vi "Main.vi"(11 "Module Admin":refnum<class "Delacor_lib_QMH_Module Admin.lvclass">) -> ()   [LabVIEW 2020, in "Navigation.lvlib"]
doc: "This template is based off of the Queued Message Handler design pattern and the Queued Message Handler project template that ships with LabVIEW.\n\nThe main difference is that the queue is private to this module and communication between modules is performed via Broadcast and Request events.\n\nRequest events are wrapped in public API methods and are handled in the Event Handling Loop (EHL) of this VI. Any module can register for Broadcast events sent by this module. The EHL generates messages based on user interface actions.\n\nThe Message Handling Loop (MHL) processes messages generated by the EHL, or by other messages. The messages are string values, so new messages can be added easily to the Message Cases case structure in the MHL. Each message cluster can also provide an optional value for Message Data, which is a variant that can be converted to whatever message-specific data is required.\n____\nHAMPEL SOFTWARE ENGINEERING v2.6.0 (2023-12-19 10:54)"
uses:
  Navigation.lvlib
  <vilib>/Delacor/Delacor QMH/Libraries/Module Admin_class/Delacor_lib_QMH_Module Admin.lvclass
  Button Manager/Control Refs.ctl
  Module Data--cluster.ctl
  <vilib>/Hampel Software Engineering/HSE Layout Manager/HSE Layout/HSE VBoxLayout/HSE VBoxLayout.lvclass
  Button Manager/Button Manager.lvclass
  Stop Argument--cluster.ctl
  <vilib>/Delacor/Delacor QMH/Libraries/Message Queue_class/Delacor_lib_QMH_Message Queue.lvclass/Delacor_lib_QMH_Message Queue.ctl
  <vilib>/Delacor/Delacor QMH/Libraries/Module Admin_class/Delacor_lib_QMH_Module Admin.lvclass/Delacor_lib_QMH_Module Admin.ctl
  Configure Argument--cluster.ctl
  Prepare Argument--cluster.ctl
  Update Navigation Argument--cluster.ctl
  Sub-VIs/Ctl Target.ctl
  Sub-VIs/ListBox Event Data.ctl
  Select Listbox Element Argument--cluster.ctl
  Set Visibility Argument--cluster.ctl
  Sub-VIs/Visibility options--enum.ctl
  Set Disabled State Argument--cluster.ctl
  Libraries/hse-libraries/Source/hse-application/hse-application.lvclass/hse-application.ctl
  Libraries/hse-libraries/Source/hse-dqmh/Controls/Module Display Scenarios.ctl
  <vilib>/Delacor/Delacor QMH/Libraries/Message Queue_class/Delacor_lib_QMH_Enqueue Message (Single).vi
  <vilib>/Delacor/Delacor QMH/Libraries/Module Admin_class/Delacor_lib_QMH_Get External Launch.vi
  Libraries/hse-libraries/Source/hse-application/HSE Application not initialized--error.vi
  Libraries/hse-libraries/Source/hse-application/hse-application__GetSingleton.vi
  <vilib>/Utility/sysdir.llb/Get System Directory.vi
  <vilib>/Utility/error.llb/Error Cluster From Error Code.vi
  <vilib>/ErrorRing/Error Ring.xnode
  <vilib>/Delacor/Delacor QMH/Libraries/Message Queue_class/Delacor_lib_QMH_Message Queue.lvclass
  Libraries/hse-libraries/Source/hse-configuration/config-ini/config-ini.lvclass
  Libraries/hse-libraries/Source/hse-application/hse-application.lvclass
  <vilib>/Hampel Software Engineering/HSE Logger/hse-logger.lvlib
  Libraries/hse-libraries/Source/hse-dqmh/hse-dqmh.lvlib
panel:
  in  "lb_sub_8":i32(listbox)
  in  "lb_sub_7":i32(listbox)
  in  "lb_sub_6":i32(listbox)
  in  "lb_sub_5":i32(listbox)
  in  "lb_sub_4":i32(listbox)
  in  "lb_sub_3":i32(listbox)
  in  "lb_sub_2":i32(listbox)
  in  "lb_sub_9":i32(listbox)
  in  "lb_sub_1":i32(listbox)
  in  "btn_top_9":bool
  in  "btn_top_8":bool
  in  "btn_top_7":bool
  in  "btn_top_6":bool
  in  "lb_sub_0":i32(listbox)
  in  "btn_top_5":bool
  in  "btn_top_4":bool
  in  "btn_top_3":bool
  in  "btn_top_2":bool
  in  "btn_top_1":bool
  in  "btn_top_0":bool
  out "error out":errorcluster
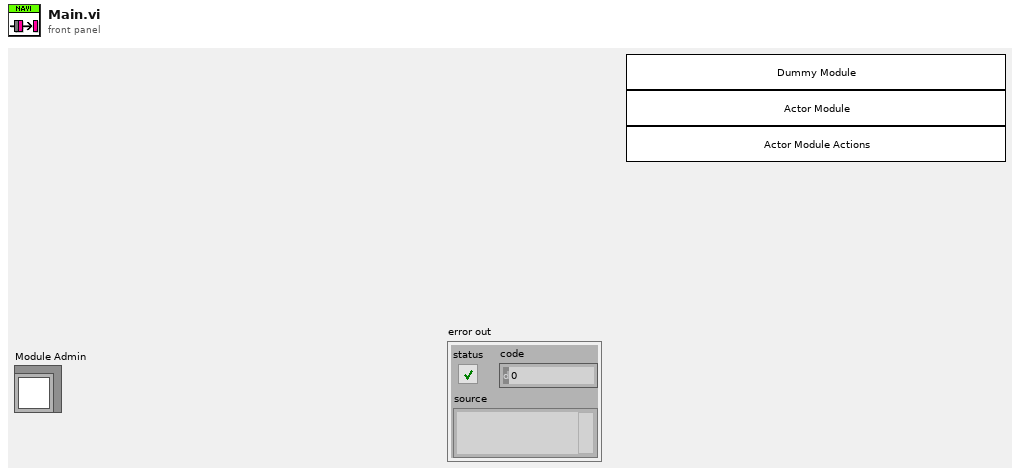
[diagram p1: front panel]
types:
  T1 = typedef "Navigation.lvlib/Button Manager.lvclass/Control Refs.ctl" = cluster{"Top Ctls":refnum<vi>[], "Sub Ctls":refnum<vi>[]}
  T2 = typedef "Navigation.lvlib/Request Events--cluster.ctl" = cluster{"Stop Module":refnum<user-event>, "Show Panel":refnum<user-event>, "Hide Panel":refnum<user-event>, "Get Module Execution Status":refnum<user-event>, "Show Diagram":refnum<user-event>, "Prepare":refnum<user-event>, "Update Navigation":refnum<user-event>, "Configure":refnum<user-event>, "Select Listbox Element":refnum<user-event>, "Set Visibility":refnum<user-event>, "Set Disabled State":refnum<user-event>}
  T3 = typedef "Navigation.lvlib/Module Data--cluster.ctl" = cluster{"VBox Layout":refnum<class "HSE VBoxLayout.lvclass">, "Button Manager":refnum<class "Button Manager.lvclass">, "Buttons Def File":path, "Subpanel VI Ref":refnum<vi>}
  T4 = enum32{"invalid lock state", "Not Locked", "Locked (No Password)", "Password-protected"}
  T5 = typedef "Navigation.lvlib/Stop Argument--cluster.ctl" = cluster{"Origin":string, "Exit via Stop Module Req?":bool, "Wait for Module to stop?":bool}
  T6 = typedef "Navigation.lvlib/Configure Argument--cluster.ctl" = cluster{"Boolean":bool}
  T7 = typedef "Navigation.lvlib/Prepare Argument--cluster.ctl" = cluster{"Boolean":bool}
  T8 = typedef "Navigation.lvlib/Update Navigation Argument--cluster.ctl" = cluster{"Ctl Target":T9, "Name":string, "Data":variant}
  T9 = typedef "Navigation.lvlib/Ctl Target.ctl" = enum16{"Top Button", "Sub ListBox"}
  T10 = typedef "Navigation.lvlib/ListBox Event Data.ctl" = cluster{"CtlRef":refnum<vi>, "NewVal":i32, "OldVal":i32}
  T11 = typedef "Navigation.lvlib/Select Listbox Element Argument--cluster.ctl" = cluster{"Name":string, "Index":i32}
  T12 = typedef "Navigation.lvlib/Set Visibility Argument--cluster.ctl" = cluster{"Control Name":string, "Visibility":T13}
  T13 = typedef "Navigation.lvlib/Visibility options--enum.ctl" = enum16{"visible", "hidden"}
  T14 = typedef "Navigation.lvlib/Set Disabled State Argument--cluster.ctl" = cluster{"Control Name":string, "Control State":enum8{"Enabled", "Disabled", "Disabled and Grayed Out"}}
  T15 = enum32{"Invalid", "Standard", "Closed", "Hidden", "Minimized", "Maximized"}
  T16 = typedef "hse-dqmh.lvlib/Module Display Scenarios.ctl" = enum16{"Stand-Alone", "Managed"}
  T17 = enum8{"Enabled", "Disabled", "Disabled and Grayed Out"}
  T18 = typedef "hse-dqmh.lvlib/System Message Source.ctl" = enum16{"module", "application", "network"}
  T19 = typedef "Navigation.lvlib/Button Manager.lvclass/Top Control.ctl" = cluster{"name":string, "caption":string, "tooltip":string, "enabled_state":string, "action":string, "display_scenario":string, "sub":T20[]}
  T20 = typedef "Navigation.lvlib/Button Manager.lvclass/Sub Control.ctl" = cluster{"name":string, "tooltip":string, "enabled_state":string, "content":string[], "retain value":bool}
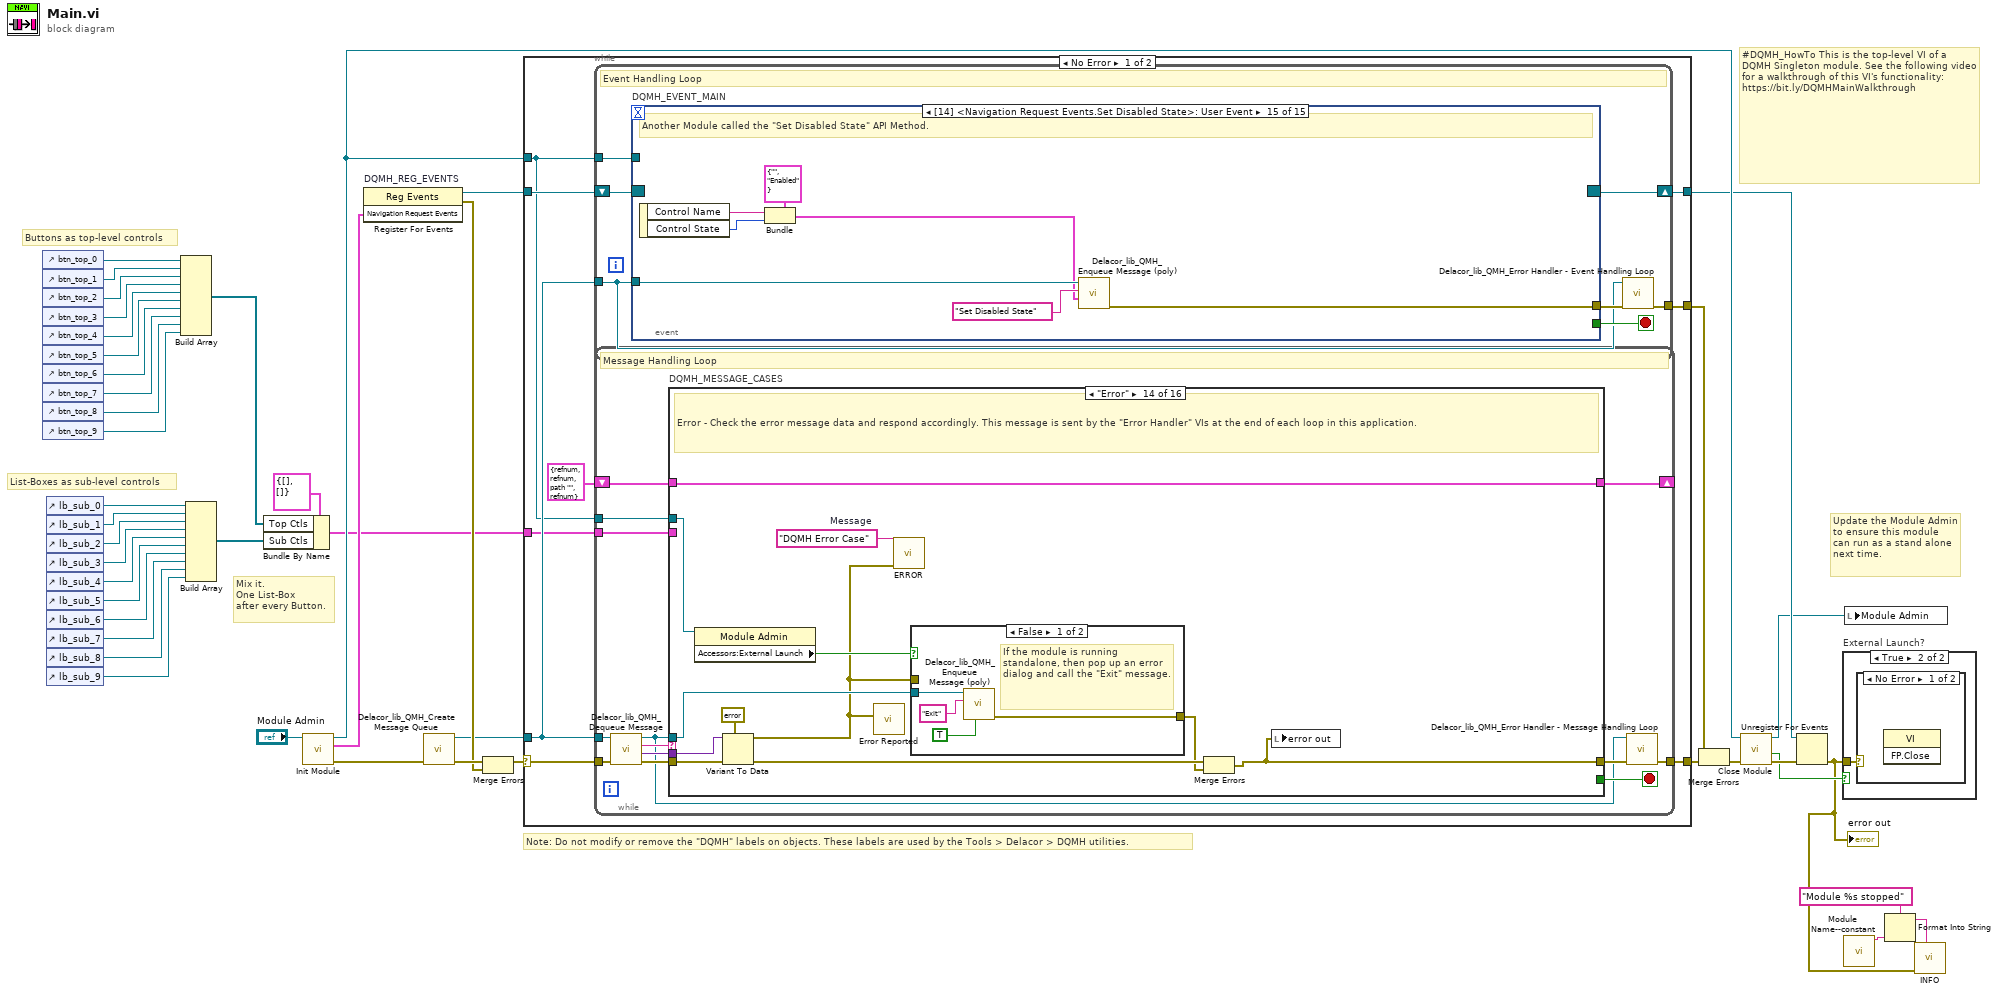
[diagram p0: block diagram]
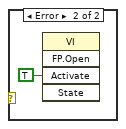
[diagram p3: hidden frame]
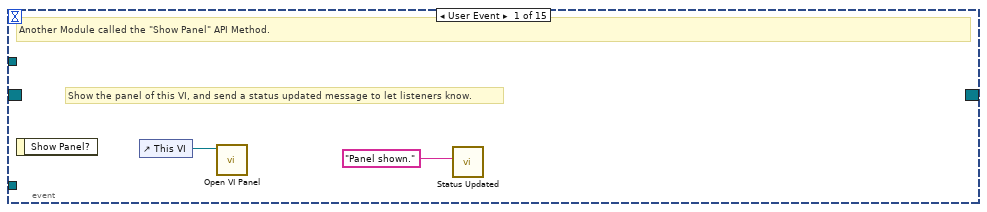
[diagram p4: hidden frame]
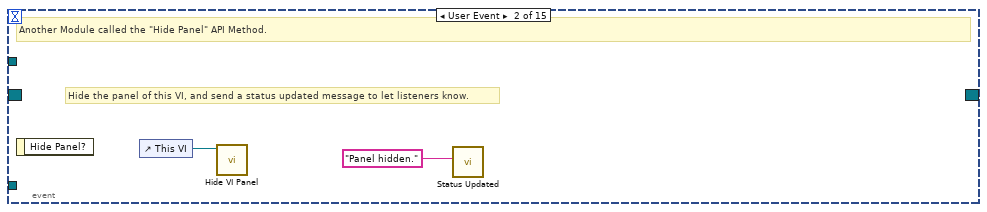
[diagram p5: hidden frame]
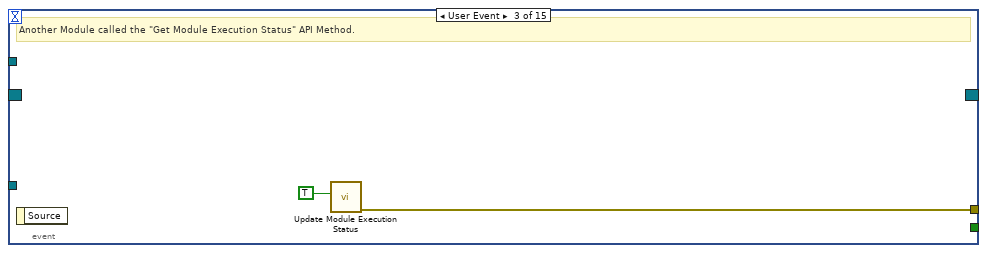
[diagram p6: hidden frame]
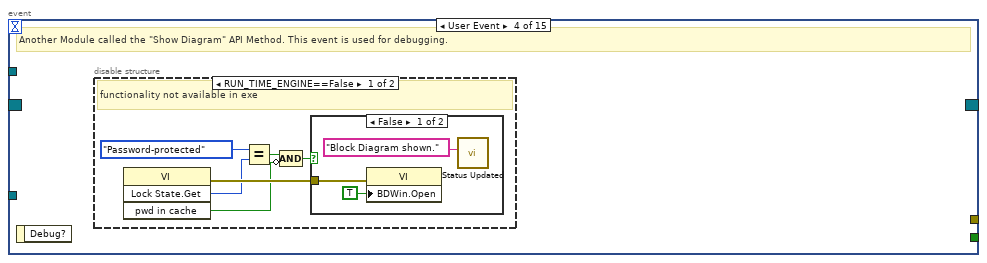
[diagram p7: hidden frame]
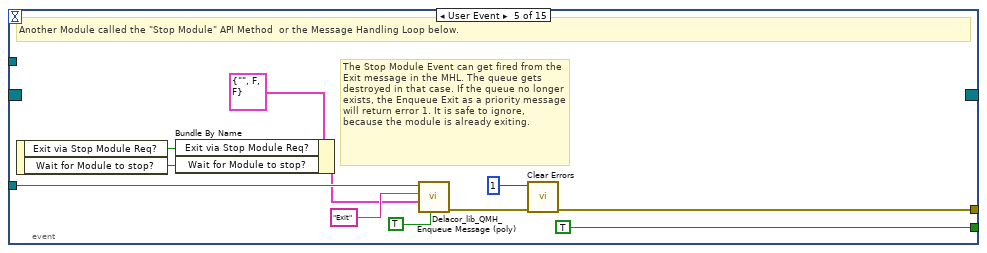
[diagram p10: hidden frame]
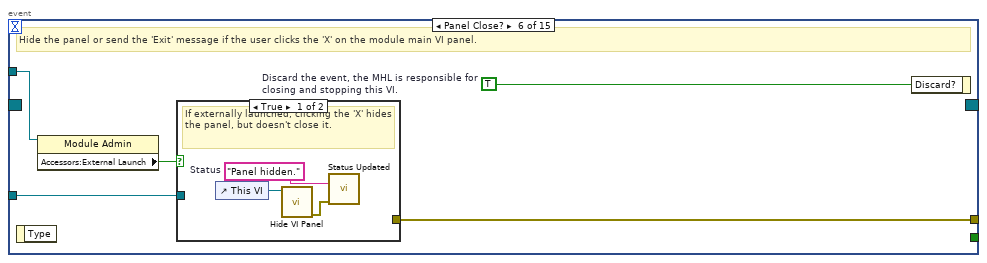
[diagram p11: hidden frame]
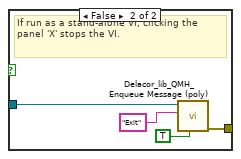
[diagram p12: hidden frame]
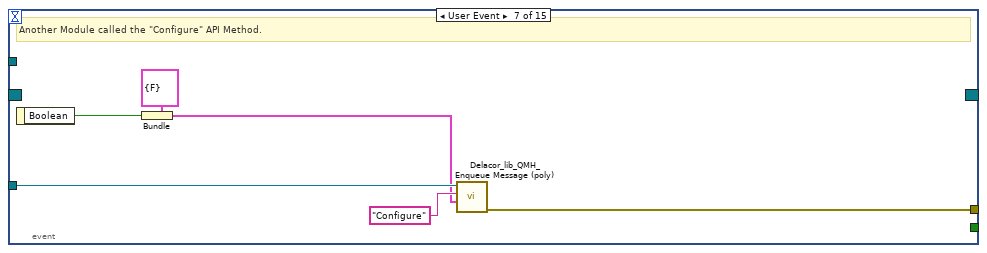
[diagram p13: hidden frame]
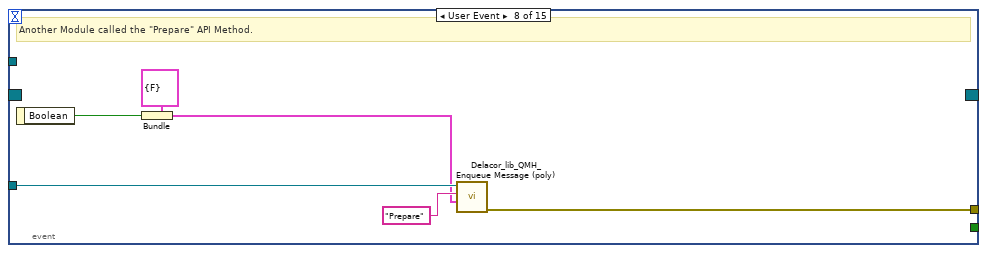
[diagram p14: hidden frame]
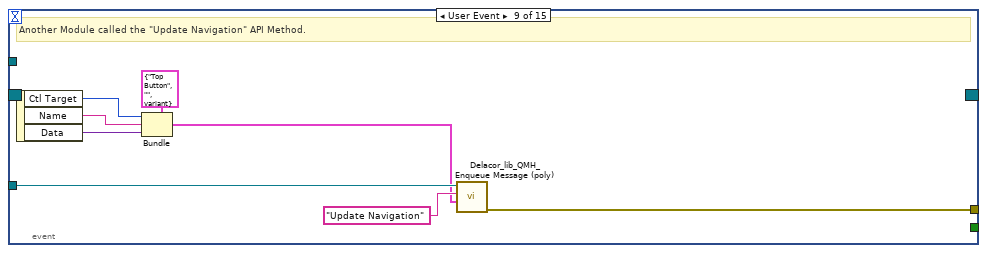
[diagram p15: hidden frame]
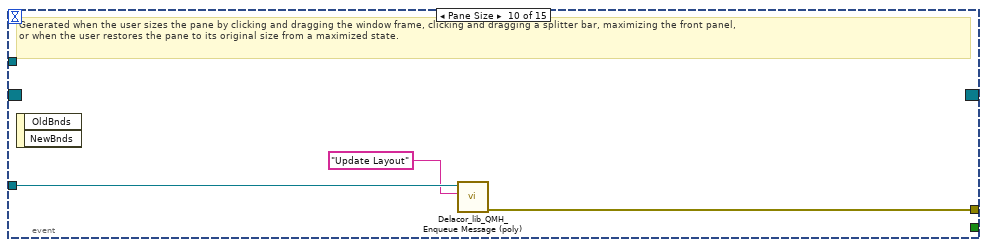
[diagram p16: hidden frame]
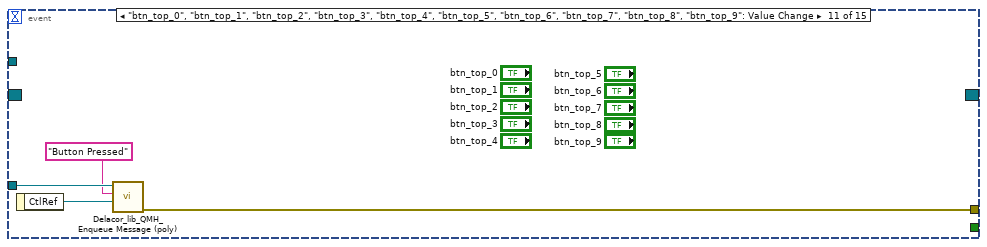
[diagram p17: hidden frame]
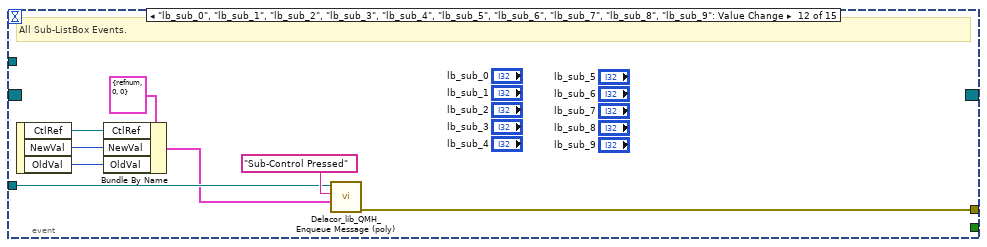
[diagram p18: hidden frame]
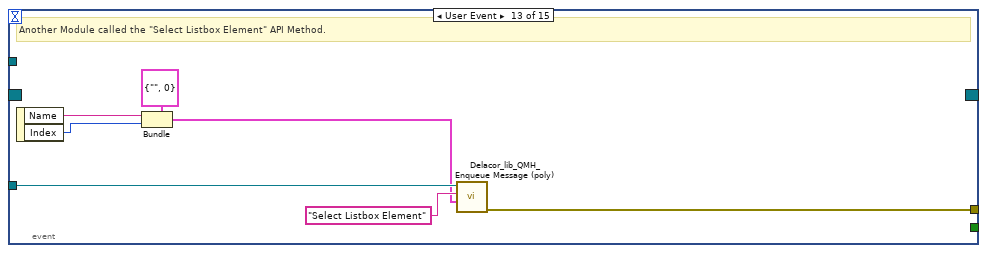
[diagram p19: hidden frame]
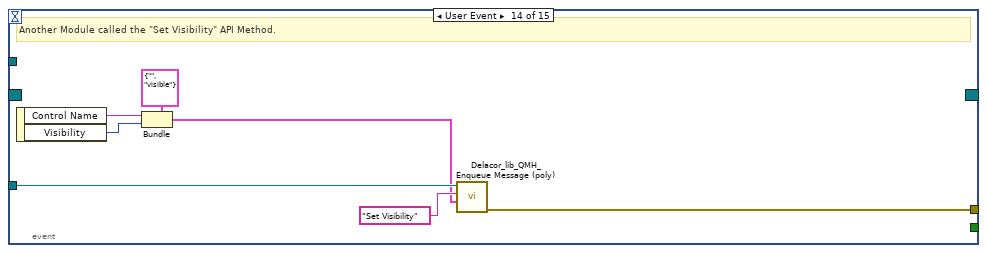
[diagram p20: hidden frame]
diagram:
  # "Mix it.\nOne List-Box\nafter every Button."
  # "List-Boxes as sub-level controls"
  # "Buttons as top-level controls"
  # "#DQMH_HowTo This is the top-level VI of a DQMH Singleton module. See the following video for a walkthrough of this VI's functionality: https://bit.ly/DQMHMainWalkthrough"
  # "Note: Do not modify or remove the \"DQMH\" labels on objects. These labels are used by the Tools > Delacor > DQMH utilities."
  # "Update the Module Admin to ensure this module can run as a stand alone next time."
  n1 = control-ref of="btn_top_0"() -> (w19:refnum<vi>)
  n2 = control-ref of="btn_top_1"() -> (w28:refnum<vi>)
  n3 = control-ref of="btn_top_2"() -> (w27:refnum<vi>)
  n4 = control-ref of="btn_top_3"() -> (w26:refnum<vi>)
  n5 = control-ref of="btn_top_4"() -> (w25:refnum<vi>)
  n6 = control-ref of="btn_top_5"() -> (w24:refnum<vi>)
  n7 = control-ref of="btn_top_6"() -> (w23:refnum<vi>)
  n8 = control-ref of="btn_top_7"() -> (w22:refnum<vi>)
  n9 = control-ref of="btn_top_8"() -> (w21:refnum<vi>)
  n10 = control-ref of="btn_top_9"() -> (w20:refnum<vi>)
  n11 = control-ref of="lb_sub_0"() -> (w18:refnum<vi>)
  n12 = control-ref of="lb_sub_1"() -> (w17:refnum<vi>)
  n13 = control-ref of="lb_sub_2"() -> (w16:refnum<vi>)
  n14 = control-ref of="lb_sub_3"() -> (w15:refnum<vi>)
  n15 = control-ref of="lb_sub_4"() -> (w14:refnum<vi>)
  n16 = control-ref of="lb_sub_5"() -> (w13:refnum<vi>)
  n17 = control-ref of="lb_sub_6"() -> (w12:refnum<vi>)
  n18 = control-ref of="lb_sub_7"() -> (w11:refnum<vi>)
  n19 = control-ref of="lb_sub_8"() -> (w10:refnum<vi>)
  n20 = control-ref of="lb_sub_9"() -> (w5:refnum<vi>)
  n21 = Build Array(w19, w28, w27, w26, w25, w24, w23, w22, w21, w20) -> (w8:refnum<vi>[])
  n22 = Build Array(w18, w17, w16, w15, w14, w13, w12, w11, w10, w5) -> (w7:refnum<vi>[])
  n23 = Bundle By Name(cluster=T1 {"Top Ctls"=[], "Sub Ctls"=[]} ("Control Refs"), "Top Ctls"=w8, "Sub Ctls"=w7) -> (w6:T1)
  n24 = call "Init Module.vi"("Singleton Module Admin in"="Module Admin") -> ("error out"=w43:errorcluster, "Navigation Request Events"=w33:T2, "Singleton Module Admin out"=w36:refnum<class "Delacor_lib_QMH_Module Admin.lvclass">)  [unwired: 8 in]
  n25 = register-events "DQMH_REG_EVENTS"(w33) -> (reference out=w34:refnum<event-registration>, error out=w37:errorcluster)  [unwired: 2 in]
  n26 = call <vilib>:"Delacor_lib_QMH_Create Message Queue.vi"("error in"=w43) -> ("error out"=w39:errorcluster, "Message Queue"=w32:refnum<class "Delacor_lib_QMH_Message Queue.lvclass">)  [unwired: 9 in]
  n27 = Merge Errors(w39, w37) -> (w38:errorcluster)
  n28 = case shown="No Error" w38 {
    selector: w38 -> [w51 w426]
    tunnel: [w53 w426] -> w44
    tunnel: [w50 w423] -> w35
    tunnel: w34 -> [w48 w423]
    tunnel: w32 -> [w47 w418]
    tunnel: [w52 _] -> w41
    tunnel: w36 -> [w46 w419]
    tunnel: w6 -> [w45 _]
    frame No Error {
      n29 = while {
        tunnel: w47 -> [w54]
        shift-right: [w57] -> w50
        shift-left: w48 -> [w58]
        tunnel: [w59] -> w52
        tunnel: w46 -> [w55]
        stop <- w56 stop-if-true
        # "Event Handling Loop"
        n30 = event "DQMH_EVENT_MAIN" shown="[14] <Navigation Request Events.Set Disabled State>: User Event" {
          selector: w58 -> [_ _ _ _ _ _ _ _ _ _ _ _ _ _ _]
          dyn-events: [_ _ _ _ _ _ _ _ _ _ _ _ _ _ _] -> w57
          timeout: _ -> [_ _ _ _ _ _ _ _ _ _ _ _ _ _ _]
          tunnel: [_ _ _ _ TRUE ("Discard?") _ _ _ _ _ _ _ _ _ _] -> w56
          tunnel: w54 -> [_ _ _ _ w82 w89 w104 w110 w118 w121 w125 w132 w140 w147 w154]
          tunnel: [_ _ w66 _ w85 w91 w99 w105 w114 w120 w124 w131 w134 w143 w148] -> w60
          tunnel: w55 -> [_ _ _ _ _ w88 _ _ _ _ _ _ _ _ _]
          event User Event {
            # "Show the panel of this VI, and send a status updated message to let listeners know."
            # "Another Module called the \"Show Panel\" API Method."
            n31 = event-data() -> ()  [unwired: 1 in, 1 out]
            n32 = control-ref of="This VI"() -> (w62:refnum<vi>)
            n33 = call "Open VI Panel.vi"("VI"=w62) -> ()  [unwired: 10 in, 1 out]
            n34 = call "Status Updated.vi"("Status"="Panel shown." ("format string")) -> ()  [unwired: 10 in, 1 out]
          }
          event User Event {
            # "Hide the panel of this VI, and send a status updated message to let listeners know."
            # "Another Module called the \"Hide Panel\" API Method."
            n35 = event-data() -> ()  [unwired: 1 in, 1 out]
            n36 = control-ref of="This VI"() -> (w64:refnum<vi>)
            n37 = call "Hide VI Panel.vi"("VI"=w64) -> ()  [unwired: 10 in, 1 out]
            n38 = call "Status Updated.vi"("Status"="Panel hidden." ("format string")) -> ()  [unwired: 10 in, 1 out]
          }
          event User Event {
            # "Another Module called the \"Get Module Execution Status\" API Method."
            n39 = event-data() -> ()  [unwired: 1 in, 1 out]
            n40 = call "Update Module Execution Status.vi"("Running?"=TRUE) -> ("error out"=w66:errorcluster)  [unwired: 10 in]
          }
          event User Event {
            # "Another Module called the \"Show Diagram\" API Method. This event is used for debugging."
            n41 = event-data() -> ()  [unwired: 1 in, 1 out]
            n42 = disable-structure shown="RUN_TIME_ENGINE==False" {
              frame condition #0 (active) {
                # "functionality not available in exe"
                n43 = invoke on="Invoke Node" class="VI" method="Lock State.Get"() -> (error out=w72:errorcluster, "Get Lock State"=w71:T4, "pwd in cache"=w68:bool)  [unwired: 4 in, 1 out]
                n44 = Equal?(x=T4."Password-protected", y=w71) -> (x = y?=w69:bool)
                n45 = Compound Arithmetic op=AND(w69, invert w68) -> (w67:bool)
                n46 = case shown="False" w67 {
                  tunnel: w72 -> [w75 _]
                  frame False {
                    n47 = property on="Property Node" class="VI"(error in=w75, "BDWin.Open"=TRUE ("Block Diagram Window:Open")) -> ()  [unwired: 1 in, 2 out]
                    n48 = call "Status Updated.vi"("Status"="Block Diagram shown." ("format string")) -> ()  [unwired: 10 in, 1 out]
                  }
                  frame True {
                    # "Password-protected VI, and the password is not in the cache. Do not show the diagram."
                  }
                }
              }
              frame condition #1 {
              }
            }
          }
          event User Event {
            # "The Stop Module Event can get fired from the Exit message in the MHL. The queue gets destroyed in that case. If the queue no longer exists, the Enqueue Exit as a priority message will return error 1. It is safe to ignore, because the module is already exiting."
            # "Another Module called the \"Stop Module\" API Method  or the Message Handling Loop below."
            n49 = event-data() -> ("Exit via Stop Module Req?"=w78:bool, "Wait for Module to stop?"=w77:bool)  [unwired: 1 in]
            n50 = Bundle By Name(cluster=T5 {"Origin"="", "Exit via Stop Module Req?"=FALSE, "Wait for Module to stop?"=FALSE} ("Stop Argument"), "Exit via Stop Module Req?"=w78, "Wait for Module to stop?"=w77) -> (w76:T5)
            n51 = call-poly <vilib>:"Delacor_lib_QMH_Enqueue Message (poly).vi"("Priority Message? (F)"=TRUE, "Message Data"=w76, "Message"="Exit", "Message Queue in"=w82) -> ("error out"=w86:errorcluster)  [unwired: 6 in, 1 out]
            n52 = call <vilib>:"Clear Errors.vi"("error in (no error)"=w86, "specific error code to clear (0: all)"=1) -> ("error out"=w85:errorcluster)  [unwired: 4 in, 1 out]
          }
          event Panel Close? {
            w90 = TRUE  # Discard the event, the MHL is responsible for closing and stopping this VI.
            # "Hide the panel or send the 'Exit' message if the user clicks the 'X' on the module main VI panel."
            n53 = event-data() -> ()  [unwired: 1 in, 1 out]
            n54 = property on="Property Node" class="Module Admin"(reference=w88) -> ("Accessors:External Launch"=w87:bool)  [unwired: 1 in, 2 out]
            n55 = case shown="True" w87 {
              tunnel: w89 -> [_ w97]
              tunnel: [_ w98] -> w91
              frame True {
                w93 = "Panel hidden."  # Status
                # "If externally launched, clicking the 'X' hides the panel, but doesn't close it."
                n56 = control-ref of="This VI"() -> (w94:refnum<vi>)
                n57 = call "Hide VI Panel.vi"("VI"=w94) -> ("error out"=w92:errorcluster)  [unwired: 10 in]
                n58 = call "Status Updated.vi"("error in (no error)"=w92, "Status"=w93) -> ()  [unwired: 9 in, 1 out]
              }
              frame False {
                # "If run as a stand-alone VI, clicking the panel 'X' stops the VI."
                n59 = call-poly <vilib>:"Delacor_lib_QMH_Enqueue Message (poly).vi"("Priority Message? (F)"=TRUE, "Message"="Exit", "Message Queue in"=w97) -> ("error out"=w98:errorcluster)  [unwired: 7 in, 1 out]
              }
            }
            n60 = event-data ("Event Filter Node")("Discard?"=w90) -> ()  [unwired: 1 in, 1 out]
          }
          event User Event {
            # "Another Module called the \"Configure\" API Method."
            n61 = event-data() -> ("Boolean"=w100:bool)  [unwired: 1 in]
            n62 = Bundle(cluster=T6 {"Boolean"=FALSE} ("Configure Argument"), "Boolean"=w100) -> (w101:T6)
            n63 = call-poly <vilib>:"Delacor_lib_QMH_Enqueue Message (poly).vi"("Message Data"=w101, "Message"="Configure", "Message Queue in"=w104) -> ("error out"=w99:errorcluster)  [unwired: 7 in, 1 out]
          }
          event User Event {
            # "Another Module called the \"Prepare\" API Method."
            n64 = event-data() -> ("Boolean"=w106:bool)  [unwired: 1 in]
            n65 = Bundle(cluster=T7 {"Boolean"=FALSE} ("Prepare Argument"), "Boolean"=w106) -> (w107:T7)
            n66 = call-poly <vilib>:"Delacor_lib_QMH_Enqueue Message (poly).vi"("Message Data"=w107, "Message"="Prepare", "Message Queue in"=w110) -> ("error out"=w105:errorcluster)  [unwired: 7 in, 1 out]
          }
          event User Event {
            # "Another Module called the \"Update Navigation\" API Method."
            n67 = event-data() -> ("Ctl Target"=w113:T9, "Name"=w112:string, "Data"=w111:variant)  [unwired: 1 in]
            n68 = Bundle(cluster=T8 {"Ctl Target"=enum."Top Button", "Name"="", "Data"=variant} ("Update Navigation Argument"), "Ctl Target"=w113, "Name"=w112, "Data"=w111) -> (w115:T8)
            n69 = call-poly <vilib>:"Delacor_lib_QMH_Enqueue Message (poly).vi"("Message Data"=w115, "Message"="Update Navigation", "Message Queue in"=w118) -> ("error out"=w114:errorcluster)  [unwired: 7 in, 1 out]
          }
          event Pane Size {
            # "Generated when the user sizes the pane by clicking and dragging the window frame, clicking and dragging a splitter bar, maximizing the front panel, \nor when the user restores the pane to its original size from a maximized state."
            n70 = event-data() -> ()  [unwired: 1 in, 2 out]
            n71 = call-poly <vilib>:"Delacor_lib_QMH_Enqueue Message (poly).vi"("Message"="Update Layout", "Message Queue in"=w121) -> ("error out"=w120:errorcluster)  [unwired: 8 in, 1 out]
          }
          event "btn_top_0", "btn_top_1", "btn_top_2", "btn_top_3", "btn_top_4", "btn_top_5", "btn_top_6", "btn_top_7", "btn_top_8", "btn_top_9": Value Change {
            n72 = event-data() -> ("CtlRef"=w122:refnum<vi>)  [unwired: 1 in]
            n73 = call-poly <vilib>:"Delacor_lib_QMH_Enqueue Message (poly).vi"("Message Data"=w122, "Message"="Button Pressed", "Message Queue in"=w125) -> ("error out"=w124:errorcluster)  [unwired: 7 in, 1 out]
          }
          event "lb_sub_0", "lb_sub_1", "lb_sub_2", "lb_sub_3", "lb_sub_4", "lb_sub_5", "lb_sub_6", "lb_sub_7", "lb_sub_8", "lb_sub_9": Value Change {
            # "All Sub-ListBox Events."
            n74 = event-data() -> ("CtlRef"=w129:refnum<vi>, "NewVal"=w128:i32, "OldVal"=w127:i32)  [unwired: 1 in]
            n75 = Bundle By Name(cluster=T10 {"CtlRef"=refnum, "NewVal"=0, "OldVal"=0} ("ListBox Event Data"), "CtlRef"=w129, "NewVal"=w128, "OldVal"=w127) -> (w126:T10)
            n76 = call-poly <vilib>:"Delacor_lib_QMH_Enqueue Message (poly).vi"("Message Data"=w126, "Message"="Sub-Control Pressed", "Message Queue in"=w132) -> ("error out"=w131:errorcluster)  [unwired: 7 in, 1 out]
          }
          event User Event {
            # "Another Module called the \"Select Listbox Element\" API Method."
            n77 = event-data() -> ("Name"=w136:string, "Index"=w135:i32)  [unwired: 1 in]
            n78 = Bundle(cluster=T11 {"Name"="", "Index"=0} ("Select Listbox Element Argument"), "Name"=w136, "Index"=w135) -> (w137:T11)
            n79 = call-poly <vilib>:"Delacor_lib_QMH_Enqueue Message (poly).vi"("Message Data"=w137, "Message"="Select Listbox Element", "Message Queue in"=w140) -> ("error out"=w134:errorcluster)  [unwired: 7 in, 1 out]
          }
          event User Event {
            # "Another Module called the \"Set Visibility\" API Method."
            n80 = event-data() -> ("Control Name"=w142:string, "Visibility"=w141:T13)  [unwired: 1 in]
            n81 = Bundle(cluster=T12 {"Control Name"="", "Visibility"=enum."visible"} ("Set Visibility Argument"), "Control Name"=w142, "Visibility"=w141) -> (w144:T12)
            n82 = call-poly <vilib>:"Delacor_lib_QMH_Enqueue Message (poly).vi"("Message Data"=w144, "Message"="Set Visibility", "Message Queue in"=w147) -> ("error out"=w143:errorcluster)  [unwired: 7 in, 1 out]
          }
          event User Event {
            # "Another Module called the \"Set Disabled State\" API Method."
            n83 = event-data() -> ("Control Name"=w150:string, "Control State"=w149:T17)  [unwired: 1 in]
            n84 = Bundle(cluster=T14 {"Control Name"="", "Control State"=enum."Enabled"} ("Set Disabled State Argument"), "Control Name"=w150, "Control State"=w149) -> (w151:T14)
            n85 = call-poly <vilib>:"Delacor_lib_QMH_Enqueue Message (poly).vi"("Message Data"=w151, "Message"="Set Disabled State", "Message Queue in"=w154) -> ("error out"=w148:errorcluster)  [unwired: 7 in, 1 out]
          }
        }
        n86 = call-dynamic "Delacor_lib_QMH_Error Handler - Event Handling Loop.vi"("error in"=w60, "Message Queue in"=w54) -> ("dup error in"=w59:errorcluster)  [unwired: 8 in, 1 out]
      }
      n87 = while {
        tunnel: w47 -> [w158]
        shift-right: [w162] -> _
        shift-left: T3 {"VBox Layout"=refnum, "Button Manager"=refnum, "Buttons Def File"=path "", "Subpanel VI Ref"=refnum} ("Data Cluster") -> [w163]
        tunnel: w51 -> [w166]
        tunnel: [w164] -> w53
        tunnel: w46 -> [w156]
        tunnel: w45 -> [w155]
        stop <- w161 stop-if-true
        # "Message Handling Loop"
        n88 = call-dynamic "Delacor_lib_QMH_Dequeue Message.vi"("error in"=w166, "Message Queue in"=w158) -> ("error out"=w165:errorcluster, "Message Data"=w159:variant, "Message"=w160:string, "Message Queue out"=w157:refnum<class "Delacor_lib_QMH_Message Queue.lvclass">)  [unwired: 6 in]
        n89 = case "DQMH_MESSAGE_CASES" shown="\"Error\"" w160 {
          selector: w160 -> [_ _ _ _ _ _ _ _ _ _ _ _ _ _ _ w405]
          tunnel: w157 -> [_ _ w200 _ _ _ _ _ _ _ _ _ _ w377 w398 _]
          tunnel: w165 -> [w182 w186 w187 w225 w227 w233 w260 w296 w309 w341 w358 w370 w372 w384 w403 w407]
          tunnel: [w168 w186 w205 w223 w227 w229 w253 w291 w303 w327 w346 w361 w372 w380 w400 w408] -> w167
          tunnel: w163 -> [w169 w185 w207 w222 w226 w231 w244 w294 w305 w331 w344 w363 w371 w379 w397 w406]
          tunnel: [w169 w185 w206 w224 w226 w230 w243 w294 w299 w331 w343 w363 w371 w379 w397 w406] -> w162
          tunnel: [_ _ _ _ _ _ _ _ _ _ _ _ _ _ w396 _] -> w161
          tunnel: w159 -> [_ _ _ _ _ _ w258 w295 w308 w340 w357 w369 _ w378 w395 _]
          tunnel: w156 -> [w174 _ _ _ _ _ _ _ _ _ _ _ _ w376 w390 _]
          tunnel: w155 -> [_ _ _ w221 _ _ w249 _ _ _ _ _ _ _ _ _]
          frame "Initialize" {
            # "Initialize - Any operation that needs to be done before the module can receive messages. Synchronize Caller Events.vi will inform Start Module.vi that the module has launched and is ready to receive messages. Module Did Init.vi will broadcast that the module initialized."
            n90 = call "Synchronize Caller Events.vi"("error in (no error)"=w182, "Singleton Module Admin in"=w174) -> ("error out"=w170:errorcluster, "Singleton Module Admin out"=w171:refnum<class "Delacor_lib_QMH_Module Admin.lvclass">)  [unwired: 8 in]
            n91 = property on="Property Node" class="Module Admin"(reference=w171) -> ("Accessors:External Launch"=w178:bool)  [unwired: 1 in, 2 out]
            n92 = Select(t=T15."Hidden" ("State"), s=w178, f=T15."Standard" ("State")) -> (s? t:f=w175:T15)
            n93 = call "Module Name--constant.vi"() -> ("Module Name"=w181:string)  [unwired: 11 in]
            n94 = property on="Property Node" class="VI"("Front Panel.Title"=w181) -> (reference out=w180:refnum<vi>, error out=w184:errorcluster)  [unwired: 2 in]
            n95 = invoke on="Invoke Node" class="VI" method="FP.Open"(reference=w180, error in=w184, "State"=w175) -> (reference out=w179:refnum<vi>, error out=w183:errorcluster)  [unwired: 2 in, 3 out]
            n96 = call "Module Name--constant.vi"() -> ("Module Name"=w172:string)  [unwired: 11 in]
            n97 = invoke on="Invoke Node" class="VI" method="FP.Center"(reference=w179, error in=w183) -> ()  [unwired: 1 in, 3 out]
            n98 = call "Module Did Init.vi"("error in (no error)"=w170, "Initialized?"=TRUE, "Origin"=w172) -> ("error out"=w168:errorcluster)  [unwired: 8 in]
          }
          frame "--- setup ---" {
            # "Separator -- The following cases handle messages specific to this Module."
          }
          frame "Configure" {
            w192 = "global" ("Section")
            # "Triggers the auto-configuration of the module."
            n99 = call "Module Name--constant.vi"() -> ("Module Name"=w190:string)  [unwired: 11 in]
            n100 = control-ref of="This VI"() -> (w193:refnum<vi>)
            n101 = call "Create Module Config.vi"("error in"=w187, "DQMH Module Name"=w190) -> ("error out"=w189:errorcluster, "config-ini out"=w188:refnum<class "config-ini.lvclass">)  [unwired: 8 in]
            n102 = call-dynamic "Read String.vi"("Section"=w192, "error in"=w189, "Key"="descriptor", "config-base in"=w188) -> ("error out"=w196:errorcluster, "Value"=w194:string, "config-base out"=w195:refnum<class "config-ini.lvclass">)  [unwired: 5 in]
            n103 = call "DQMH System Message - Add to Run-Time Menu.vi"("Module Descriptor"=w194, "Main VI Reference"=w193) -> ("Payload"=w198:variant, "Identifier"=w199:string, "Source"=w197:T18)  [unwired: 7 in]
            n104 = property class="VI"("Front Panel.Title"=w194) -> ()  [unwired: 2 in, 2 out]
            n105 = call "System Message.vi"("Sys. Msg. Source"=w197, "Payload"=w198, "Identifier"=w199) -> ()  [unwired: 8 in, 1 out]
            n106 = call-dynamic "Read String.vi"("Section"=w192, "error in"=w196, "Key"="buttons_def", "config-base in"=w195) -> ("error out"=w210:errorcluster, "Value"=w209:string)  [unwired: 5 in, 1 out]
            n107 = call "hse-application_GetApplicationPaths.vi"("error in"=w210) -> ("error out"=w202:errorcluster, "Config/Unit Directory"=w208:path)  [unwired: 4 in, 5 out]
            n108 = Build Path(base path=w208, name or relative path=w209) -> (appended path=w203:path)
            n109 = disable-structure shown="Enabled" {
              disable-tunnel: w202 -> [w215 w216]
              disable-tunnel: [w214 w216] -> w201
              disable-tunnel: w200 -> [w213 _]
              frame Disabled {
                w212 = "Prepare"  # Message
                # "Call own prepare event"
                n110 = call-poly <vilib>:"Delacor_lib_QMH_Enqueue Message (poly).vi"("error in"=w215, "Message"=w212, "Message Queue in"=w213) -> ("error out"=w214:errorcluster)  [unwired: 7 in, 1 out]
              }
              frame Enabled {
              }
            }
            n111 = Bundle By Name(cluster=w207, "Buttons Def File"=w203) -> (w206:T3)
            n112 = call <vilib>:"DEBUG.vi"("Message"="Module Navigation configured", "error in"=w201) -> ("error out"=w205:errorcluster)  [unwired: 9 in]
          }
          frame "Prepare" {
            # "Prepares the frontpanel for display."
            n113 = Unbundle By Name(w222) -> ("Buttons Def File"=w217:path)
            n114 = control-ref of="Pane"() -> (w220:refnum<vi>)
            n115 = call "Prepare - Initialize Objects.vi"("Buttons Def File"=w217, "error in (no error)"=w225, "Pane"=w220, "Control Refs"=w221) -> ("error out"=w223:errorcluster, "HSE VBox Layout"=w218:refnum<class "HSE VBoxLayout.lvclass">, "Button Manager out"=w219:refnum<class "Button Manager.lvclass">)  [unwired: 5 in]
            n116 = Bundle By Name(cluster=w222, "Button Manager"=w219, "VBox Layout"=w218) -> (w224:T3)
          }
          frame "--- Module Specific ---" {
            # "Separator -- The following cases handle messages specific to this Module."
          }
          frame "Update Layout" {
            w228 = 1055  # specific error code to clear (0: all)
            # "#todo currently the \"Update Layout\" event is triggered at load time\nbefore the \"Configure\" and \"Prepare\" cases are executed.\n--> Find a way to solve this more elegantly."
            # "Resizes and repositions the controls on the FP after the pane was resized."
            n117 = in-place {
              in-place-border: w233 -> [w236]
              in-place-border: [w239] -> w232
              n118 = in-place-cluster #1(w231) -> ("VBox Layout"=w238:refnum<class "HSE VBoxLayout.lvclass">)
              n119 = control-ref of="Pane"() -> (w234:refnum<vi>)
              n120 = call-dynamic "Pane Update.vi"("error in"=w236, "Pane"=w234, "HSE Layout in"=w238) -> ("error out"=w235:errorcluster, "HSE Layout out"=w237:refnum<class "HSE VBoxLayout.lvclass">)  [unwired: 7 in]
              n121 = call-dynamic "Update.vi"("error in"=w235, "HSE VBoxLayout in"=w237) -> ("error out"=w239:errorcluster, "HSE VBoxLayout out"=w240:refnum<class "HSE VBoxLayout.lvclass">)  [unwired: 8 in]
              n122 = in-place-cluster #1("VBox Layout"=w240) -> (w230:T3)
            }
            n123 = call <vilib>:"Clear Errors.vi"("error in (no error)"=w232, "specific error code to clear (0: all)"=w228) -> ("error out"=w229:errorcluster)  [unwired: 4 in, 1 out]
          }
          frame "Button Pressed" {
            # "A Navigation Button was pressed."
            n124 = Variant To Data(error in=w260, type=refnum<vi> refnum ("CtlRef"), Variant=w258) -> (data=w251:refnum<vi>, error out=w248:errorcluster)
            n125 = Unbundle By Name(w244) -> ("Button Manager"=w252:refnum<class "Button Manager.lvclass">)
            n126 = Unbundle By Name(w244) -> ("VBox Layout"=w245:refnum<class "HSE VBoxLayout.lvclass">)
            n127 = Unbundle By Name(w249) -> ("Sub Ctls"=w247:refnum<vi>[])
            n128 = call-dynamic "Get Object by Ctl-Ref.vi"("Ctl Ref in"=w251, "Button Manager in"=w252) -> ("error out"=w263:errorcluster, "Button Object"=w250:T19, "Sub-Ctl Ref"=w246:refnum<vi>)  [unwired: 5 in, 2 out]
            n129 = Unbundle By Name(w250) -> ("sub"=w242:T20[], "name"=w254:string, "action"=w255:string, "display_scenario"=w257:string)
            n130 = call "Hide not selected Sub-Ctls.vi"("sub"=w242, "error in"=w263, "Sub-Ctls"=w247, "Sub-Ctl Visible"=w246, "VBox Layout"=w245) -> ("error out"=w262:errorcluster, "VBox Layout"=w241:refnum<class "HSE VBoxLayout.lvclass">)  [unwired: 5 in]
            n131 = call "Button Pressed.vi"("error in (no error)"=w262, "action"=w255, "name"=w254) -> ("error out"=w261:errorcluster)  [unwired: 8 in]
            n132 = case "Wich display scenario?" shown="\"Managed\"" w257 {
              tunnel: w255 -> [_ w270 w277]
              tunnel: w261 -> [w264 w271 w278]
              tunnel: [w264 w267 w276] -> w256
              frame "None", Default {
                # "Do not display a module."
              }
              frame "Stand-Alone" {
                # "Display a module stand-alone."
                n133 = call "Get Module Path.vi"("error in"=w271, "Module Name"=w270) -> ("error out"=w268:errorcluster, "module path"=w266:path)  [unwired: 8 in]
                n134 = control-ref of="This Application"() -> (w265:refnum<vi>)
                n135 = call "Request UI Display--helper.vi"("This Application"=w265, "error in (no error)"=w268, "Display Scenario"=Module_Display_Scenarios."Stand-Alone", "Module DQMH Path"=w266) -> ("error out"=w267:errorcluster)  [unwired: 7 in]
              }
              frame "Managed" {
                # "Display a module in the UI Manager."
                n136 = call "Get Module Path.vi"("error in"=w278, "Module Name"=w277) -> ("error out"=w275:errorcluster, "module path"=w274:path)  [unwired: 8 in]
                n137 = control-ref of="This Application"() -> (w272:refnum<vi>)
                n138 = call "Request UI Display--helper.vi"("This Application"=w272, "error in (no error)"=w275, "Display Scenario"=Module_Display_Scenarios."Managed", "Module DQMH Path"=w274) -> ("error out"=w276:errorcluster)  [unwired: 7 in]
              }
            }
            n139 = Bundle By Name(cluster=w244, "VBox Layout"=w241) -> (w243:T3)
            n140 = Merge Errors(w248, w256) -> (w253:errorcluster)
          }
          frame "Sub-Control Pressed" {
            # "A Navigation Button was pressed."
            n141 = Variant To Data(error in=w296, type=T10 {"CtlRef"=refnum, "NewVal"=0, "OldVal"=0} ("ListBox Event Data"), Variant=w295) -> (data=w292:T10, error out=w290:errorcluster)
            n142 = Unbundle By Name(w294) -> ("Button Manager"=w286:refnum<class "Button Manager.lvclass">)
            n143 = Unbundle By Name(w292) -> ("CtlRef"=w285:refnum<vi>, "NewVal"=w287:i32, "OldVal"=w289:i32)
            n144 = call-dynamic "Get Object by Ctl-Ref.vi"("Ctl Ref in"=w285, "Button Manager in"=w286) -> ("error out"=w283:errorcluster, "Button Object"=w284:T19, "Sub-Ctl Ref"=w280:refnum<vi>)  [unwired: 5 in, 2 out]
            n145 = Unbundle By Name(w284) -> ("sub"=w281:T20[])
            n146 = Index Array(array=w281) -> (element=w279:T20)  [unwired: 1 in]
            n147 = call "Retain Or Reset Sub Value.vi"("ListBox in"=w280, "error in (no error)"=w283, "sub object"=w279) -> ("error out"=w282:errorcluster)  [unwired: 8 in]
            n148 = Unbundle By Name(w279) -> ("name"=w288:string)
            n149 = call "Sub-Control Pressed.vi"("error in (no error)"=w282, "OldVal"=w289, "NewVal"=w287, "Name"=w288) -> ("error out"=w297:errorcluster)  [unwired: 7 in]
            n150 = Merge Errors(w290, w297) -> (w291:errorcluster)
          }
          frame "Update Navigation" {
            # "Send information for updating the Navigation to some state."
            n151 = Variant To Data(error in=w309, type=T8 {"Ctl Target"=enum."Top Button", "Name"="", "Data"=variant} ("Update Navigation Argument"), Variant=w308) -> (data=w306:T8, error out=w302:errorcluster)
            n152 = Unbundle By Name(w306) -> ("Ctl Target"=w301:T9, "Name"=w300:string, "Data"=w304:variant)
            n153 = case shown="\"Sub ListBox\"" w301 {
              tunnel: w305 -> [w312 w326]
              tunnel: w304 -> [_ w324]
              tunnel: w300 -> [w310 w316]
              tunnel: [w312 w326] -> w299
              tunnel: [w311 w317] -> w298
              frame "Top Button" {
                # "Do something usefull."
                # "Manipulate a top-level Button."
                n154 = Unbundle By Name(w312) -> ("Button Manager"=w313:refnum<class "Button Manager.lvclass">)
                n155 = call-dynamic "Get Object by Name.vi"("Name"=w310, "Button Manager in"=w313) -> ("error out"=w311:errorcluster)  [unwired: 6 in, 3 out]
              }
              frame "Sub ListBox" {
                w315 = refnum<vi> refnum  # ListBox
                # "manipulate a sub-level ListBox (select row)."
                n156 = Unbundle By Name(w326) -> ("Button Manager"=w325:refnum<class "Button Manager.lvclass">)
                n157 = Variant To Data(type=0, Variant=w324) -> (data=w314:i32, error out=w322:errorcluster)  [unwired: 1 in]
                n158 = call-dynamic "Get Object by Name.vi"("error in"=w322, "Name"=w316, "Button Manager in"=w325) -> ("error out"=w319:errorcluster, "Ctl Ref"=w321:refnum<vi>)  [unwired: 5 in, 2 out]
                n159 = To More Specific Class(target class=w315, reference=w321, error in=w319) -> (specific class reference=w320:refnum<vi>, error out=w318:errorcluster)
                n160 = property class="LstBox"(reference=w320, error in=w318, "Val(Sgnl)"=w314) -> (error out=w317:errorcluster)  [unwired: 1 out]
              }
            }
            n161 = Merge Errors(w302, w298) -> (w303:errorcluster)
          }
          frame "Select Listbox Element" {
            w332 = refnum<vi> refnum  # ListBox
            # "Selects a listbox element identified by name and index"
            n162 = Variant To Data(error in=w341, type=T11 {"Name"="", "Index"=0} ("Select Listbox Element Argument"), Variant=w340) -> (data=w338:T11, error out=w328:errorcluster)
            n163 = Unbundle By Name(w331) -> ("Button Manager"=w337:refnum<class "Button Manager.lvclass">)
            n164 = Unbundle By Name(w338) -> ("Name"=w329:string, "Index"=w330:i32)
            n165 = call-dynamic "Get Object by Name.vi"("error in"=w328, "Name"=w329, "Button Manager in"=w337) -> ("error out"=w334:errorcluster, "Ctl Ref"=w336:refnum<vi>)  [unwired: 5 in, 2 out]
            n166 = To More Specific Class(target class=w332, reference=w336, error in=w334) -> (specific class reference=w335:refnum<vi>, error out=w333:errorcluster)
            n167 = property class="LstBox"(reference=w335, error in=w333, "Val(Sgnl)"=w330) -> (error out=w327:errorcluster)  [unwired: 1 out]
          }
          frame "Set Visibility" {
            # "Shows or hides a  control"
            n168 = Variant To Data(error in=w358, type=T12 {"Control Name"="", "Visibility"=enum."visible"} ("Set Visibility Argument"), Variant=w357) -> (data=w355:T12, error out=w352:errorcluster)
            n169 = Unbundle By Name(w344) -> ("VBox Layout"=w349:refnum<class "HSE VBoxLayout.lvclass">, "Button Manager"=w354:refnum<class "Button Manager.lvclass">)
            n170 = Unbundle By Name(w355) -> ("Control Name"=w353:string, "Visibility"=w351:T13)
            n171 = call-dynamic "Get Object by Name.vi"("error in"=w352, "Name"=w353, "Button Manager in"=w354) -> ("error out"=w347:errorcluster, "Ctl Ref"=w348:refnum<vi>)  [unwired: 5 in, 2 out]
            n172 = Equal?(x=w351, y=Visibility_options--enum."visible") -> (x = y?=w345:bool)
            n173 = call-dynamic "Set Ctl Visibility.vi"("error in"=w347, "Visible?"=w345, "Ctl Refnum"=w348, "HSE Layout in"=w349) -> ("error out"=w346:errorcluster, "HSE Layout out"=w342:refnum<class "HSE VBoxLayout.lvclass">)  [unwired: 5 in, 1 out]
            n174 = Bundle By Name(cluster=w344, "VBox Layout"=w342) -> (w343:T3)
          }
          frame "Set Disabled State" {
            # "Enables or disables a control identified by <b>Control Name</b>"
            n175 = Variant To Data(error in=w370, type=T14 {"Control Name"="", "Control State"=enum."Enabled"} ("Set Disabled State Argument"), Variant=w369) -> (data=w367:T14, error out=w360:errorcluster)
            n176 = Unbundle By Name(w363) -> ("Button Manager"=w366:refnum<class "Button Manager.lvclass">)
            n177 = Unbundle By Name(w367) -> ("Control Name"=w362:string, "Control State"=w359:T17)
            n178 = call-dynamic "Get Object by Name.vi"("error in"=w360, "Name"=w362, "Button Manager in"=w366) -> ("error out"=w364:errorcluster, "Ctl Ref"=w365:refnum<vi>)  [unwired: 5 in, 2 out]
            n179 = property class="Ctl"(reference=w365, error in=w364, "DisabledEnum"=w359) -> (error out=w361:errorcluster)  [unwired: 1 out]
          }
          frame "--- Exit and Error Handling---" {
            # "Separator - The following cases handle errors and exit messages."
          }
          frame "Error" {
            w373 = "DQMH Error Case"  # Message
            # "Error - Check the error message data and respond accordingly. This message is sent by the \"Error Handler\" VIs at the end of each loop in this application."
            n180 = property on="Property Node" class="Module Admin"(reference=w376) -> ("Accessors:External Launch"=w375:bool)  [unwired: 1 in, 2 out]
            n181 = Variant To Data(error in=w384, type=errorcluster {"status"=FALSE, "code"=0, "source"=""} ("error constant"), Variant=w378) -> (data=w374:errorcluster, error out=w382:errorcluster)
            n182 = call "Error Reported.vi"("Error"=w374) -> ()  [unwired: 10 in, 1 out]
            n183 = call <vilib>:"ERROR.vi"("Message"=w373, "error in"=w374) -> ()  [unwired: 9 in, 1 out]
            n184 = case shown="False" w375 {
              tunnel: [w388 _] -> w381
              tunnel: w377 -> [w387 _]
              tunnel: w374 -> [_ _]
              frame False {
                # "If the module is running standalone, then pop up an error dialog and call the \"Exit\" message."
                n185 = call-poly <vilib>:"Delacor_lib_QMH_Enqueue Message (poly).vi"("Priority Message? (F)"=TRUE, "Message"="Exit", "Message Queue in"=w387) -> ("error out"=w388:errorcluster)  [unwired: 7 in, 1 out]
              }
              frame True {
                # "If the module was launched externally, calling the Error Reported broadcast VI is the only action performed by the \"Error\" message. The module's caller can then process the error appropriately."
              }
            }
            n186 = Merge Errors(w382, w381) -> (w380:errorcluster)
            n187 = local write "error out"(w380) -> ()
          }
          frame "Exit" {
            w394 = 91  # 91: not all Exit messages will have an argument
            w396 = TRUE  # Stop the VI
            # "Release the message queue reference"
            # "#CodeNeeded - Add any required cleanup code here"
            # "Exit - Exit the application."
            n188 = Variant To Data(error in=w403, type=T5 {"Origin"="", "Exit via Stop Module Req?"=FALSE, "Wait for Module to stop?"=FALSE} ("Stop Argument"), Variant=w395) -> (data=w392:T5, error out=w399:errorcluster)
            n189 = call <vilib>:"Clear Errors.vi"("error in (no error)"=w399, "specific error code to clear (0: all)"=w394) -> ("error out"=w402:errorcluster)  [unwired: 4 in, 1 out]
            n190 = control-ref of="This VI"() -> (w391:refnum<vi>)
            n191 = call-dynamic "Delacor_lib_QMH_Release Message Queue.vi"("error in"=w402, "Message Queue"=w398) -> ("error out"=w401:errorcluster)  [unwired: 9 in]
            n192 = call "Handle Exit.vi"("Stop Argument"=w392, "Admin in"=w390, "VI reference"=w391) -> ("error out"=w389:errorcluster)  [unwired: 7 in, 1 out]
            n193 = Merge Errors(w401, w389) -> (w400:errorcluster)
            n194 = call "Error Reported.vi"("Error"=w400) -> ()  [unwired: 10 in, 1 out]
          }
          frame Default {
            # "'Default' case only runs if there is a message that isn't defined in any of the other cases.  Output a programming error."
            n195 = call "Module Name--constant.vi"() -> ("Module Name"=w404:string)  [unwired: 11 in]
            n196 = xnode "Error Ring"("parameter 0"=w405, "parameter 1"=w404) -> ("error out"=w409:errorcluster)
            n197 = Merge Errors(w407, w409) -> (w408:errorcluster)
          }
        }
        n198 = call-dynamic "Delacor_lib_QMH_Error Handler - Message Handling Loop.vi"("error in"=w167, "Message Queue in"=w157) -> ("dup error in"=w164:errorcluster)  [unwired: 8 in, 1 out]
      }
    }
    frame Error {
      # "Synchronize Caller Events.vi will inform Start Module.vi that the module has launched and will let the code calling Start Module.vi register for broadcasts and would permit the caller receive the broadcast that an error occurred at launch time."
      n199 = call-dynamic "Delacor_lib_QMH_Release Message Queue.vi"("Message Queue"=w418) -> ()  [unwired: 10 in, 1 out]
      n200 = call "Synchronize Caller Events.vi"("Singleton Module Admin in"=w419) -> ("error out"=w424:errorcluster)  [unwired: 9 in, 1 out]
      n201 = call "Module Name--constant.vi"() -> ("Module Name"=w422:string)  [unwired: 11 in]
      n202 = Format Into String(format string="An error occurred during initialization. %s is no longer running.", w422) -> (resulting string=w420:string)  [unwired: 2 in, 1 out]
      n203 = Merge Errors(w426, w424) -> (w425:errorcluster)
      n204 = call "Error Reported.vi"("Additional Information"=w420, "Error"=w425) -> ()  [unwired: 9 in, 1 out]
    }
  }
  n205 = Merge Errors(w41, w44) -> (w40:errorcluster)
  n206 = call "Close Module.vi"("error in (no error)"=w40, "Module Admin in"=w36) -> ("error out"=w42:errorcluster, "External Launch"=w29:bool, "Module Admin out"=w30:refnum<class "Delacor_lib_QMH_Module Admin.lvclass">)  [unwired: 7 in]
  n207 = Unregister For Events(event registration refnum=w35, error in=w42) -> (error out=w1:errorcluster)
  "error out" <- w1
  n208 = case "External Launch?" shown="True" w29 {
    tunnel: w1 -> [_ w427]
    frame False {
    }
    frame True {
      n209 = case shown="No Error" w427 {
        frame No Error {
          n210 = invoke on="Invoke Node" class="VI" method="FP.Close"() -> ()  [unwired: 3 in, 3 out]
        }
        frame Error {
          n211 = invoke on="Invoke Node" class="VI" method="FP.Open"("Activate"=TRUE ("Activate?")) -> ()  [unwired: 4 in, 5 out]
        }
      }
    }
  }
  n212 = call "Module Name--constant.vi"() -> ("Module Name"=w2:string)  [unwired: 11 in]
  n213 = local write "Module Admin"(w30) -> ()
  n214 = Format Into String(format string="Module %s stopped", w2) -> (resulting string=w3:string)  [unwired: 2 in, 1 out]
  n215 = call <vilib>:"INFO.vi"("Message"=w3, "error in"=w1) -> ()  [unwired: 9 in, 1 out]
